vi "Read Resource.vi"(8 "error in (no error)":errorcluster, 11 "io configuration in":refnum<class "io configuration.lvclass">) -> (0 "error out":errorcluster, 2 "Resource":string, 3 "io configuration out":refnum<class "io configuration.lvclass">)   [LabVIEW 2017, in "io configuration.lvclass"]
uses:
  io configuration.lvclass
  io configuration.lvclass/io configuration.ctl
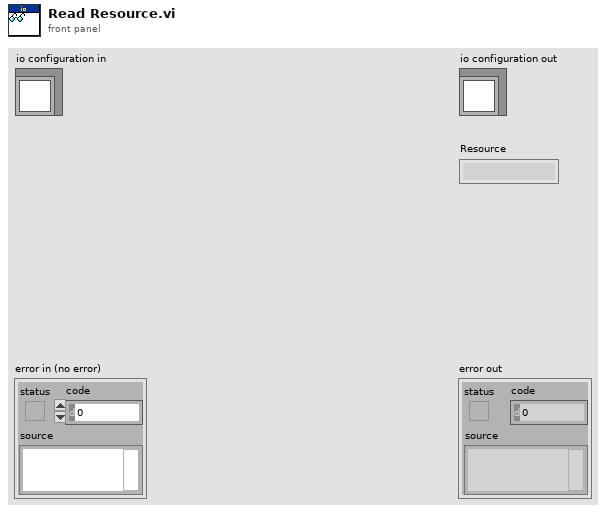
[diagram p1: front panel]
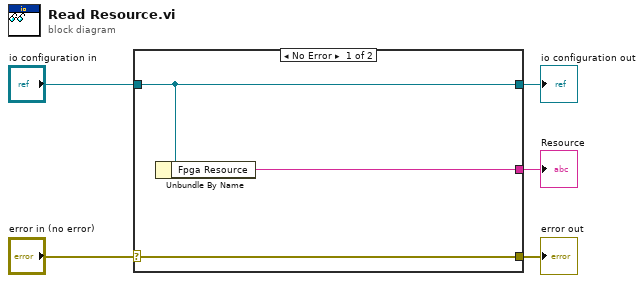
[diagram p0: block diagram]
diagram:
  n1 = case shown="No Error" "error in (no error)" {
    selector: "error in (no error)" -> [w8 w9]
    tunnel: [w8 w9] -> w4
    tunnel: [w7 w10] -> w2
    tunnel: "io configuration in" -> [w7 w10]
    tunnel: [w6 _] -> w1
    frame No Error {
      n2 = Unbundle By Name(w7) -> ("Fpga Resource"=w6:string)
    }
    frame Error {
    }
  }
  "error out" <- w4
  "io configuration out" <- w2
  "Resource" <- w1
